vi "DI Test.vi"() -> ()   [LabVIEW 2018]
uses:
  <vilib>/DAQmx/write.llb/DAQmx Write (Digital 1D Bool NChan 1Samp 1Line).vi
  <vilib>/DAQmx/read.llb/DAQmx Read (Digital 1D Bool NChan 1Samp 1Line).vi
  <vilib>/DAQmx/create/channels.llb/DAQmx Create Channel (DO-Digital Output).vi
  <vilib>/DAQmx/miscellaneous.llb/DAQmx Fill In Error Info.vi
panel:
  out "data 2":bool[](array[boolean]) caption="数据"
  out "data":bool[](array[boolean]) caption="数据"
  in  "initial value 2":bool caption="初始值"
  in  "initial value":bool caption="初始值"
  in  "error in 2":errorcluster caption="错误输入"
  out "error out":errorcluster caption="错误输出"
  in  "error in":errorcluster caption="错误输入"
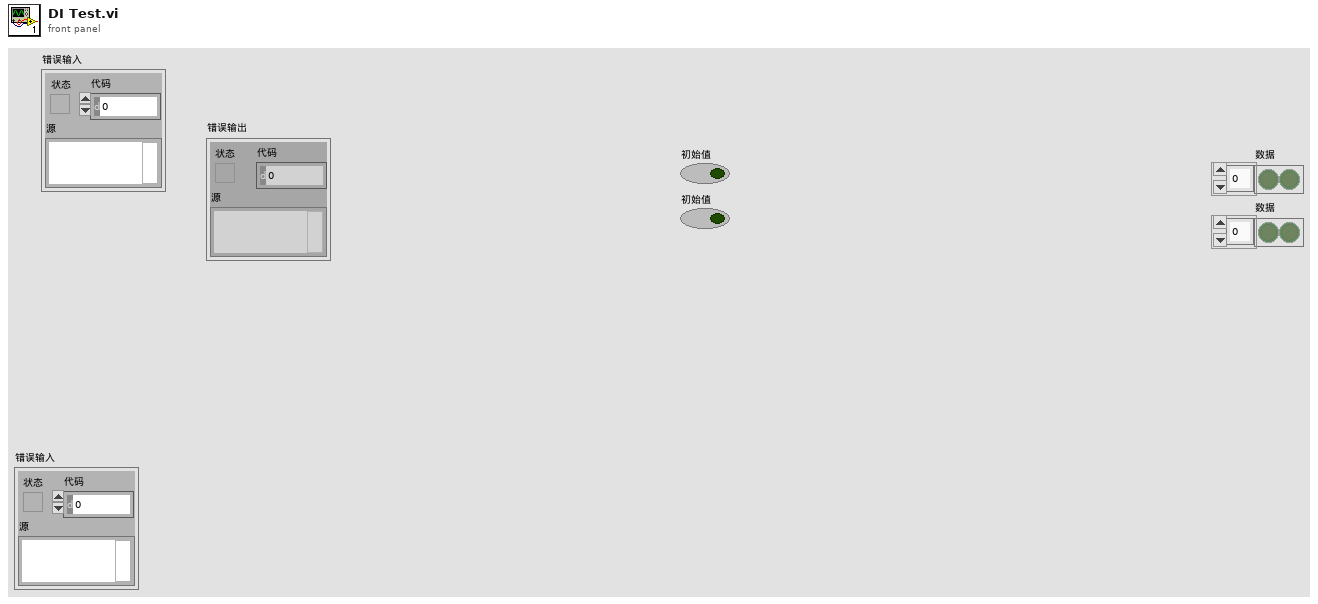
[diagram p1: front panel]
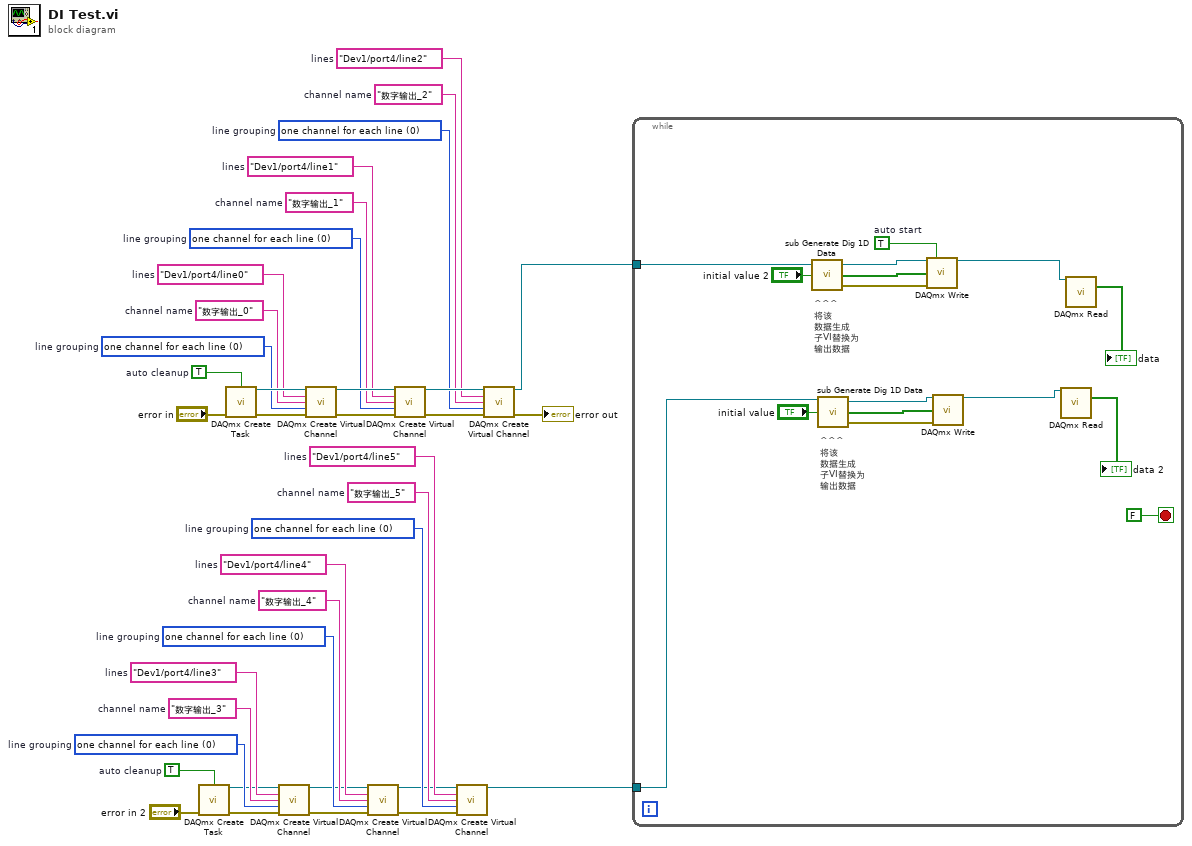
[diagram p0: block diagram]
diagram:
  w17 = 0 items=["one channel for each line", "one channel for all lines"]  # line grouping
  w18 = "数字输出_5"  # channel name
  w16 = "Dev1/port4/line5"  # lines
  w12 = 0 items=["one channel for each line", "one channel for all lines"]  # line grouping
  w13 = "数字输出_4"  # channel name
  w11 = "Dev1/port4/line4"  # lines
  w7 = 0 items=["one channel for each line", "one channel for all lines"]  # line grouping
  w8 = "数字输出_3"  # channel name
  w6 = "Dev1/port4/line3"  # lines
  w4 = TRUE  # auto cleanup
  w22 = 0 items=["one channel for each line", "one channel for all lines"]  # line grouping
  w21 = "数字输出_2"  # channel name
  w23 = "Dev1/port4/line2"  # lines
  w27 = 0 items=["one channel for each line", "one channel for all lines"]  # line grouping
  w26 = "数字输出_1"  # channel name
  w28 = "Dev1/port4/line1"  # lines
  w32 = 0 items=["one channel for each line", "one channel for all lines"]  # line grouping
  w31 = "数字输出_0"  # channel name
  w33 = "Dev1/port4/line0"  # lines
  w35 = TRUE  # auto cleanup
  n1 = call <vilib>:"DAQmx Create Task.vi"("auto cleanup"=w4, "error in"="error in 2") -> ("task out"=w5:refnum<k21>, "error out"=w3:errorcluster)  [unwired: 12 in]
  n2 = call <vilib>:"DAQmx Create Task.vi"("auto cleanup"=w35, "error in"="error in") -> ("task out"=w34:refnum<k21>, "error out"=w36:errorcluster)  [unwired: 12 in]
  n3 = call-poly <vilib>:"DAQmx Create Virtual Channel.vi"("task in"=w5, "lines"=w6, "name to assign"=w8, "line grouping"=w7, "error in"=w3) -> ("task out"=w10:refnum<k21>, "error out"=w9:errorcluster)  [unwired: 9 in]
  n4 = call-poly <vilib>:"DAQmx Create Virtual Channel.vi"("task in"=w34, "lines"=w33, "name to assign"=w31, "line grouping"=w32, "error in"=w36) -> ("task out"=w29:refnum<k21>, "error out"=w30:errorcluster)  [unwired: 9 in]
  n5 = call-poly <vilib>:"DAQmx Create Virtual Channel.vi"("task in"=w10, "lines"=w11, "name to assign"=w13, "line grouping"=w12, "error in"=w9) -> ("task out"=w15:refnum<k21>, "error out"=w14:errorcluster)  [unwired: 9 in]
  n6 = call-poly <vilib>:"DAQmx Create Virtual Channel.vi"("task in"=w29, "lines"=w28, "name to assign"=w26, "line grouping"=w27, "error in"=w30) -> ("task out"=w24:refnum<k21>, "error out"=w25:errorcluster)  [unwired: 9 in]
  n7 = call-poly <vilib>:"DAQmx Create Virtual Channel.vi"("task in"=w15, "lines"=w16, "name to assign"=w18, "line grouping"=w17, "error in"=w14) -> ("task out"=w1:refnum<k21>)  [unwired: 9 in, 1 out]
  n8 = call-poly <vilib>:"DAQmx Create Virtual Channel.vi"("task in"=w24, "lines"=w23, "name to assign"=w21, "line grouping"=w22, "error in"=w25) -> ("task out"=w19:refnum<k21>, "error out"=→"error out":errorcluster)  [unwired: 9 in]
  n9 = while {
    tunnel: w19 -> [w45]
    tunnel: w1 -> [w44]
    stop <- FALSE stop-if-true
    w53 = TRUE  # auto start
    # "^^^\n将该\n数据生成\n子VI替换为\n输出数据"
    # "^^^\n将该\n数据生成\n子VI替换为\n输出数据"
    n10 = call <vilib>:"sub Generate Dig 1D Data.vi"("initial value"="initial value 2", "task in"=w45) -> ("error out"=w52:errorcluster, "Data"=w51:bool[], "task out"=w50:refnum<k21>)  [unwired: 1 in]
    n11 = call <vilib>:"sub Generate Dig 1D Data.vi"("initial value"="initial value", "task in"=w44) -> ("error out"=w48:errorcluster, "Data"=w49:bool[], "task out"=w47:refnum<k21>)  [unwired: 1 in]
    n12 = call-poly <vilib>:"DAQmx Write.vi"("task/channels in"=w50, "auto start"=w53, "data"=w51, "error in"=w52) -> ("task out"=w41:refnum<k21>)  [unwired: 9 in, 2 out]
    n13 = call-poly <vilib>:"DAQmx Write.vi"("task/channels in"=w47, "data"=w49, "error in"=w48) -> ("task out"=w39:refnum<k21>)  [unwired: 10 in, 2 out]
    n14 = call-poly <vilib>:"DAQmx Read.vi"("task/channels in"=w39) -> ("data"=→"data 2":bool[])  [unwired: 12 in, 2 out]
    n15 = call-poly <vilib>:"DAQmx Read.vi"("task/channels in"=w41) -> ("data"=→"data":bool[])  [unwired: 12 in, 2 out]
  }
